vi "KE_Measure_Vf.vi"(5 "Settle Delay":u32, 6 "Samples":i32=1, 7 "Keep On":bool, 8 "error in (no error)":errorcluster, 9 "Compliance":dbl=0.1, 10 "Current(A)":dbl, 11 "KE_In":refnum<visa-resource-name>) -> (0 "error out":errorcluster, 1 "Vf":dbl format="%0.2f", 3 "KE_Out":refnum<visa-resource-name>)   [LabVIEW 2012]
uses:
  <instrlib>/Keithley 24XX/Public/Data/Read (Multiple Points).vi
  <vilib>/Analysis/baseanly.llb/Mean (DBL).vi
  <instrlib>/Keithley 24XX/Keithley 24XX.lvlib
  <vilib>/Analysis/NI_AALBase.lvlib
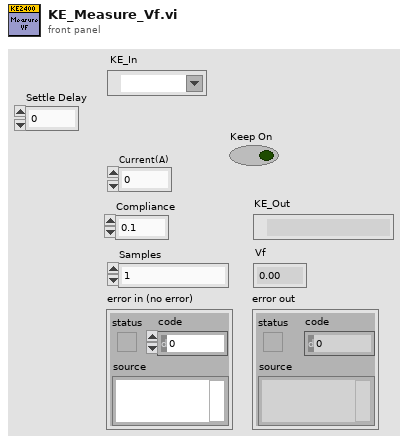
[diagram p1: front panel]
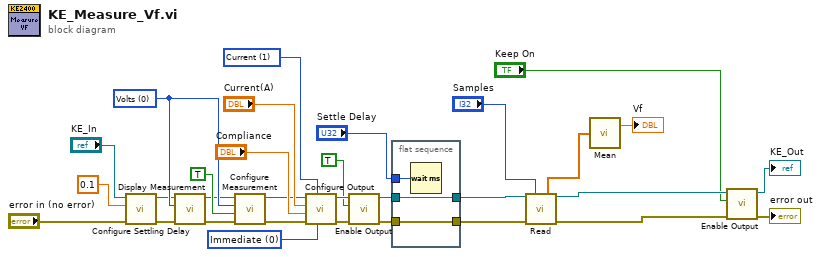
[diagram p0: block diagram]
diagram:
  w7 = u16 0 items=["Immediate", "Triggered"] ("Output Type  (0: Immediate)")
  w19 = u16 0 items=["Volts", "Current", "Resistance"] ("Function (0: Volts)")
  w8 = u16 1 items=["Voltage", "Current"] ("Source Mode  (0: Voltage)")
  n1 = call <instrlib>:"Configure Settling Delay.vi"("error in (no error)"="error in (no error)", "Manual Settling Delay (0 sec)"=0.1, "VISA resource name"="KE_In") -> ("error out"=w13:errorcluster, "VISA resource name out"=w16:refnum<visa-resource-name>)  [unwired: 7 in]
  n2 = call <instrlib>:"Display Measurement.vi"("error in (no error)"=w13, "Displayed Measurement (0: Voltage)"=w19, "VISA resource name"=w16) -> ("error out"=w17:errorcluster, "VISA resource name out"=w18:refnum<visa-resource-name>)  [unwired: 7 in]
  n3 = call <instrlib>:"Configure Measurement.vi"("error in (no error)"=w17, "Enable Auto Range (T:Enable)"=TRUE, "Function (0: Volts)"=w19, "VISA resource name"=w18) -> ("error out"=w10:errorcluster, "VISA resource name out"=w11:refnum<visa-resource-name>)  [unwired: 6 in]
  n4 = call <instrlib>:"Configure Output.vi"("Output Type  (0: Immediate)"=w7, "Source Mode  (0: Voltage)"=w8, "error in (no error)"=w10, "Compliance  Level (0.1)"="Compliance", "Output Level (0)"="Current(A)", "VISA resource name"=w11) -> ("error out"=w30:errorcluster, "VISA resource name out"=w31:refnum<visa-resource-name>)  [unwired: 4 in]
  n5 = call <instrlib>:"Enable Output.vi"("error in (no error)"=w30, "Enable Output (T: Enable)"=TRUE, "VISA resource name"=w31) -> ("error out"=w4:errorcluster, "VISA resource name out"=w3:refnum<visa-resource-name>)  [unwired: 7 in]
  n6 = flat-sequence {
    tunnel: "Settle Delay" -> [w34]
    tunnel: [w33] -> w5
    tunnel: w4 -> [w33]
    tunnel: w3 -> [w32]
    tunnel: [w32] -> w2
    frame #0 {
      n7 = Wait (ms)(milliseconds to wait=w34) -> ()  [unwired: 1 out]
    }
  }
  n8 = call-poly <instrlib>:"Read.vi"("VISA resource name"=w2, "Sample Count (1)"="Samples", "error in (no error)"=w5) -> ("Voltage"=w9:sgl[], "VISA resource name out"=w24:refnum<visa-resource-name>, "error out"=w23:errorcluster)  [unwired: 6 in, 4 out]
  n9 = call-poly <vilib>:"Mean.vi"("X"=w9) -> ("mean"=→"Vf":dbl)  [unwired: 1 out]
  n10 = call <instrlib>:"Enable Output.vi"("error in (no error)"=w23, "Enable Output (T: Enable)"="Keep On", "VISA resource name"=w24) -> ("error out"=→"error out":errorcluster, "VISA resource name out"=→"KE_Out":refnum<visa-resource-name>)  [unwired: 7 in]
